vi "save python lineouts.vi"(10 "Path":path, 11 "Point Grey Camera in":refnum<class "Point Grey Camera.lvclass">) -> ()   [LabVIEW 2020, in "Point Grey Camera.lvclass"]
uses:
  Point Grey Camera.lvclass
  Point Grey Camera.lvclass/Point Grey Camera.ctl
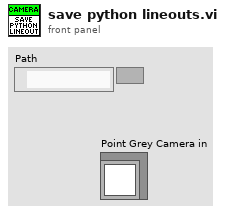
[diagram p1: front panel]
types:
  T1 = typedef "OnOffTypeDef.ctl" = enum16{"off", "on"}
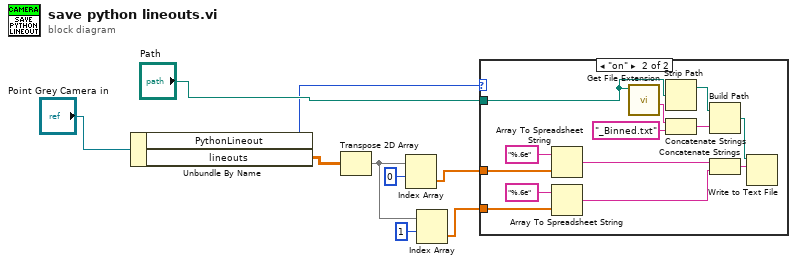
[diagram p0: block diagram]
diagram:
  n1 = Unbundle By Name("Point Grey Camera in") -> ("PythonLineout"=w8:T1, "lineouts"=w6:dbl[][])
  n2 = Transpose 2D Array(2D array=w6) -> (transposed array=w3:dbl[][])
  n3 = Index Array(array=w3, index (row)=0) -> (element=w4:dbl[])  [unwired: 1 in]
  n4 = Index Array(array=w3, index (row)=1) -> (element=w1:dbl[])  [unwired: 1 in]
  n5 = case shown="\"on\"" w8 {
    tunnel: "Path" -> [_ w17]
    tunnel: w4 -> [_ w11]
    tunnel: w1 -> [_ w10]
    frame "off", Default {
    }
    frame "on" {
      n6 = Array To Spreadsheet String(array=w11, 3:"%.6e" ("format string")) -> (spreadsheet string=w14:string)  [unwired: 1 in]
      n7 = Array To Spreadsheet String(array=w10, 3:"%.6e" ("format string")) -> (spreadsheet string=w13:string)  [unwired: 1 in]
      n8 = call <vilib>:"Get File Extension.vi"("file"=w17) -> ("filename without extension"=w21:string)  [unwired: 6 in, 4 out]
      n9 = Strip Path(path=w17) -> (stripped path=w19:path)  [unwired: 1 out]
      n10 = Concatenate Strings(w21, "_Binned.txt" ("string")) -> (w20:string)
      n11 = Build Path(base path=w19, name or relative path=w20) -> (appended path=w22:path)
      n12 = Concatenate Strings(w14, w13) -> (w12:string)
      n13 = Write to Text File(file (use dialog)=w22, text=w12) -> ()  [unwired: 2 in, 3 out]
    }
  }
